vi "MQTT Publisher.vi"() -> ()   [LabVIEW 2021]
uses:
  <vilib>/LabVIEW Open Source Project/MQTT Control Packets/Control Packets/CONNECT/ConnectFlags -- cluster.ctl
  <vilib>/LabVIEW Open Source Project/MQTT Connection/MQTT_Base/Base Class/MQTT_Base.lvclass/MQTT_Base.ctl
  <vilib>/LabVIEW Open Source Project/Connection/Connection.TCP/Connection.TCP.lvclass
  C:/Program Files (x86)/National Instruments/LabVIEW 2021/vi.lib/LabVIEW Open Source Project/Connection/Connection/Connection.lvclass
  <vilib>/LabVIEW Open Source Project/MQTT Client/Client class/Client.lvclass
  C:/Program Files (x86)/National Instruments/LabVIEW 2021/vi.lib/LabVIEW Open Source Project/MQTT Connection/MQTT_Base/Base Class/MQTT_Base.lvclass
  <vilib>/LabVIEW Open Source Project/MQTT Control Packets/Control Packets/PUBLISH/PUBLISH.lvclass
  <vilib>/LabVIEW Open Source Project/MQTT Connection/MQTT_Base/Base Class/MQTT_Base.lvclass
  <vilib>/LabVIEW Open Source Project/MQTT Control Packets/Control Packets/CONNECT/CONNECT.lvclass
panel:
  out "Connected?":bool
  out "Published":bool
  in  "Topic":string
  out "Data Chart":dbl(graph)
  out "Data":dbl format="%#_4g"
  in  "Time Target (s)":dbl=1.0 format="%#_6ps"
  in  "remote port (1883)":u16=1883
  in  "address (localhost)":string="localhost"
  in  "STOP":bool
  # "MQTT Publisher"
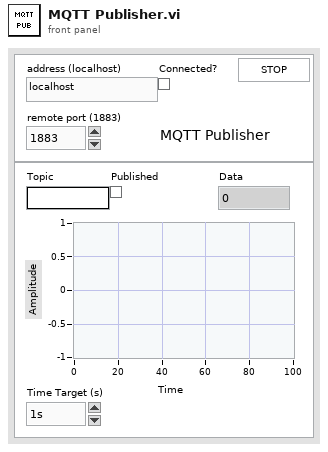
[diagram p1: front panel]
types:
  T1 = enum32{"Invalid", "Standard", "Closed", "Hidden", "Minimized", "Maximized"}
  T2 = enum32{"invalid app kind", "Development System", "Run Time System", "Student Edition", "Embedded LabVIEW", "Evaluation", "Custom"}
  T3 = typedef "MQTT_Control_Packets.lvlib/CONNECT.lvclass/ConnectFlags -- cluster.ctl" = cluster{"Reserved":bool, "Clean Session":bool, "Will Flag":bool, "Will QoS 1":bool, "Will QoS 2":bool, "Will Retain":bool, "Password Flag":bool, "User Name Flag":bool}
  T4 = cluster{"Will Topic":string, "Will Message":string, "Username":string, "Password":string}
  T5 = cluster{"Core":cluster{"Current VI Reference":refnum<vi>, "Close Panel on Exit?":bool}, "Connected?":bool, "Published?":bool, "Dummy Data":dbl}
  T6 = cluster{"Current VI Reference":refnum<vi>, "Close Panel on Exit?":bool}
  T7 = typedef "MQTT Base.lvlib/MQTT_Base.lvclass/Public Events -- cluster.ctl" = cluster{"Stop Event":refnum<user-event>, "Error Event":refnum<user-event>, "Inbound Message":refnum<user-event>}
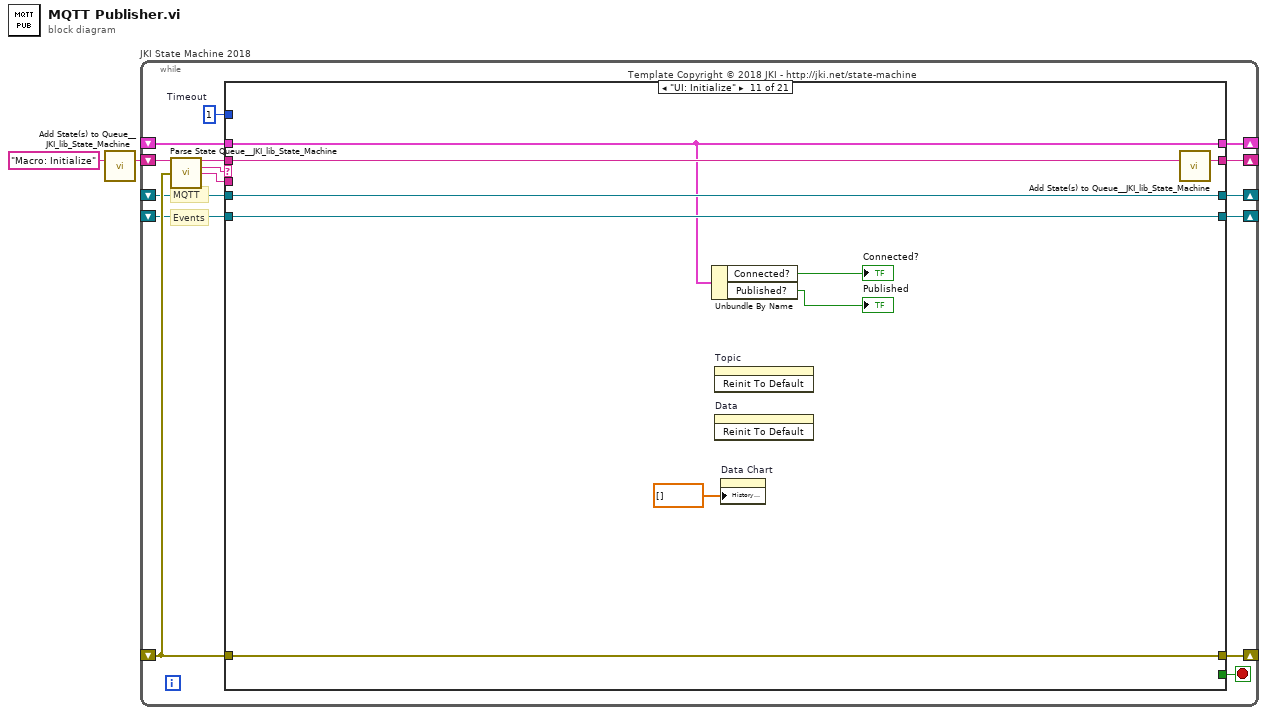
[diagram p0: block diagram]
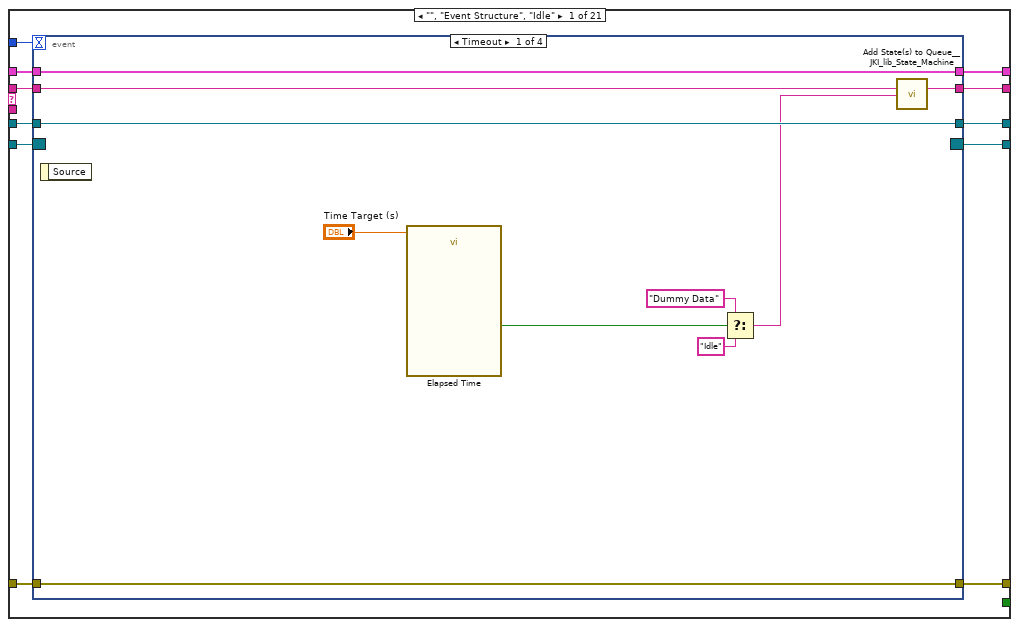
[diagram p2: hidden frame]
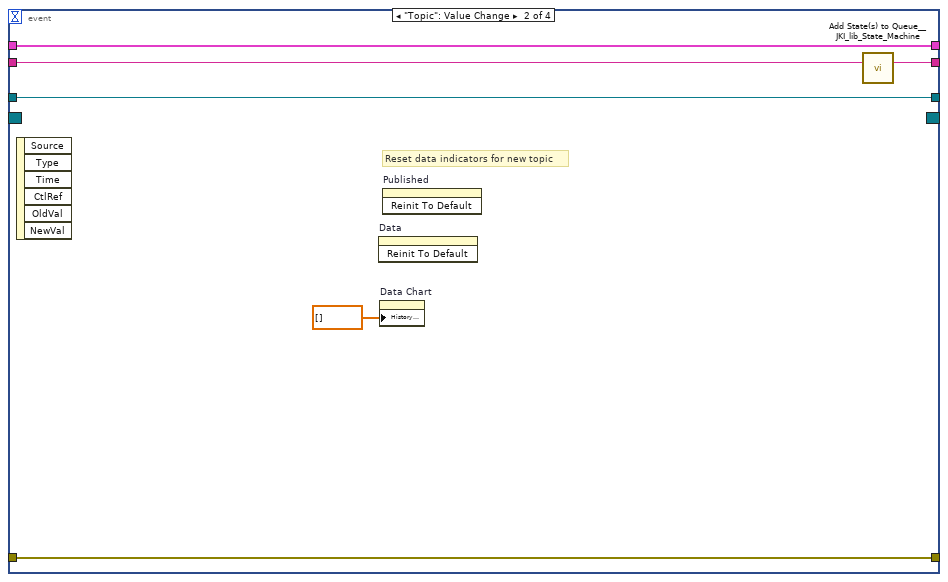
[diagram p3: hidden frame]
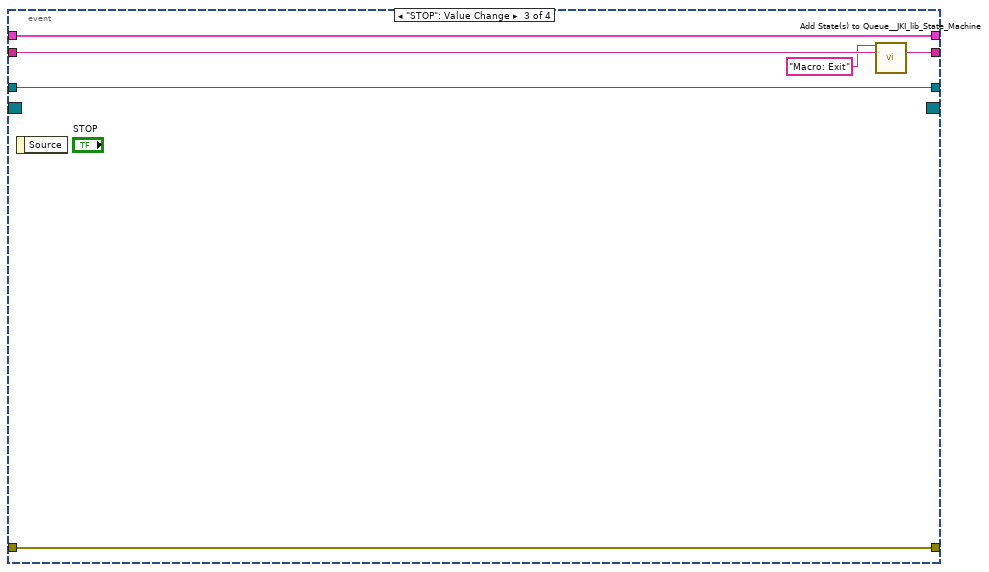
[diagram p4: hidden frame]
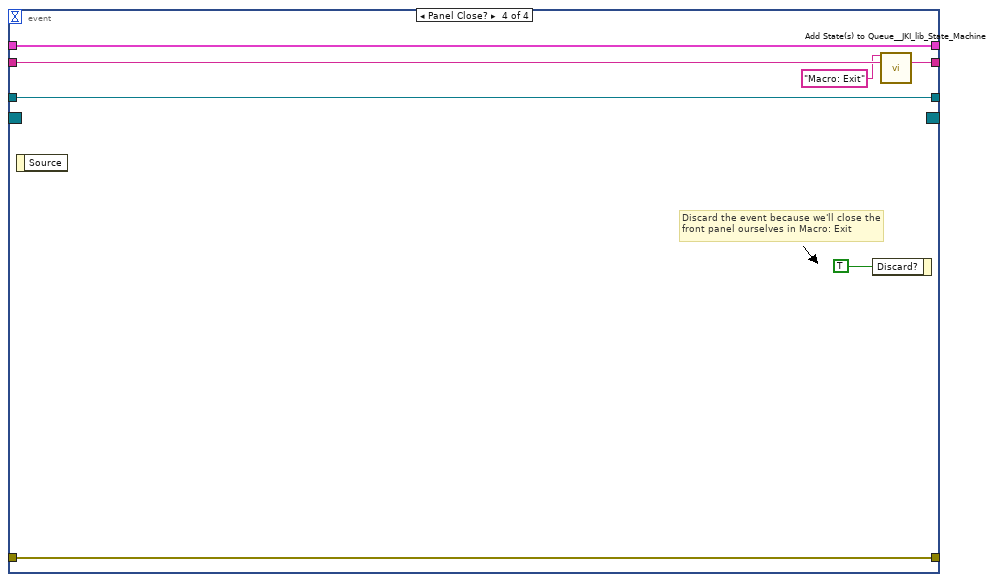
[diagram p5: hidden frame]
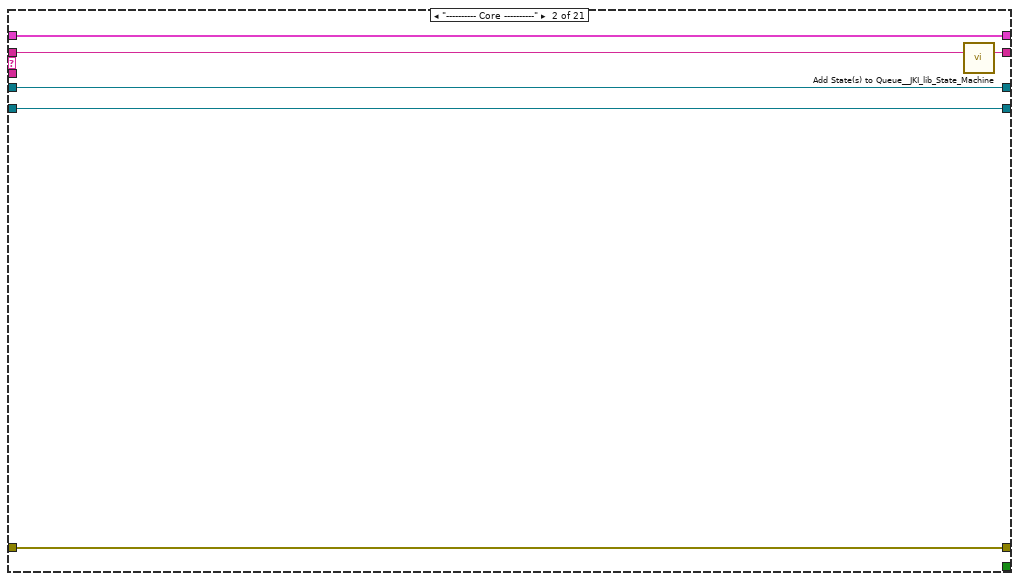
[diagram p6: hidden frame]
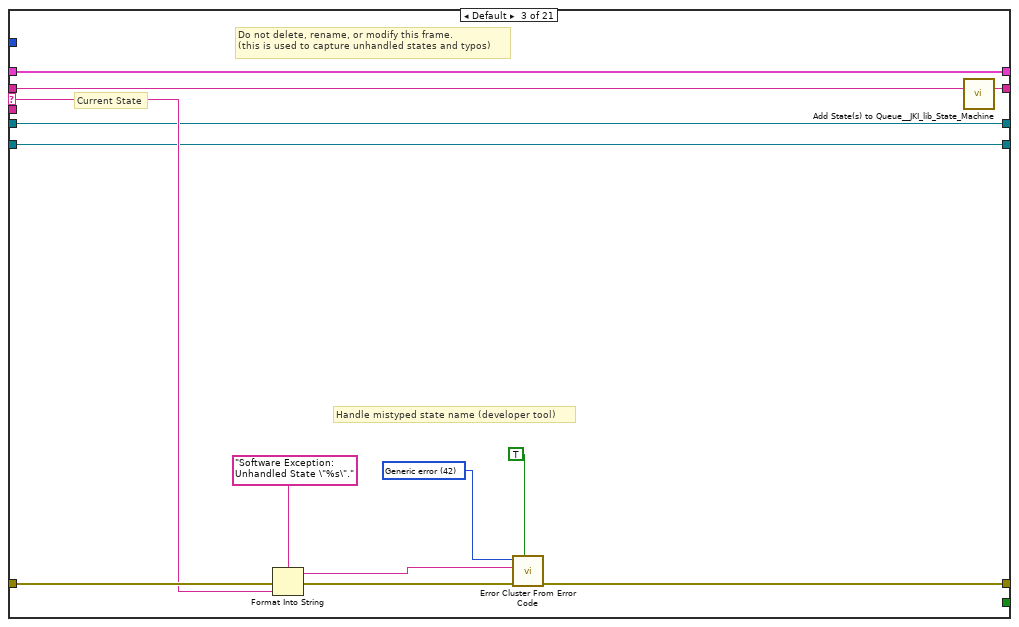
[diagram p7: hidden frame]
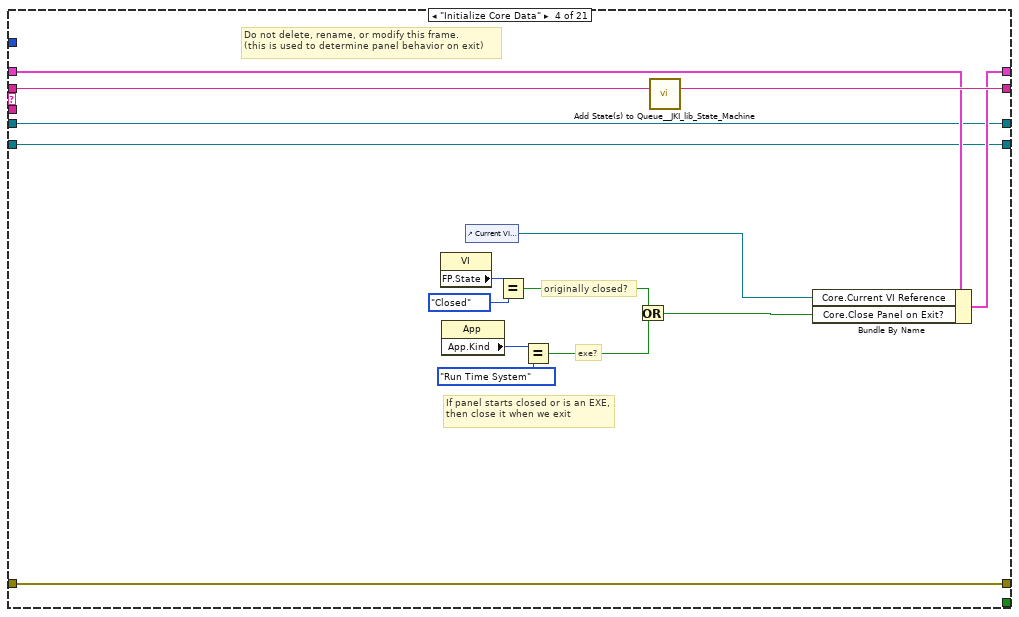
[diagram p8: hidden frame]
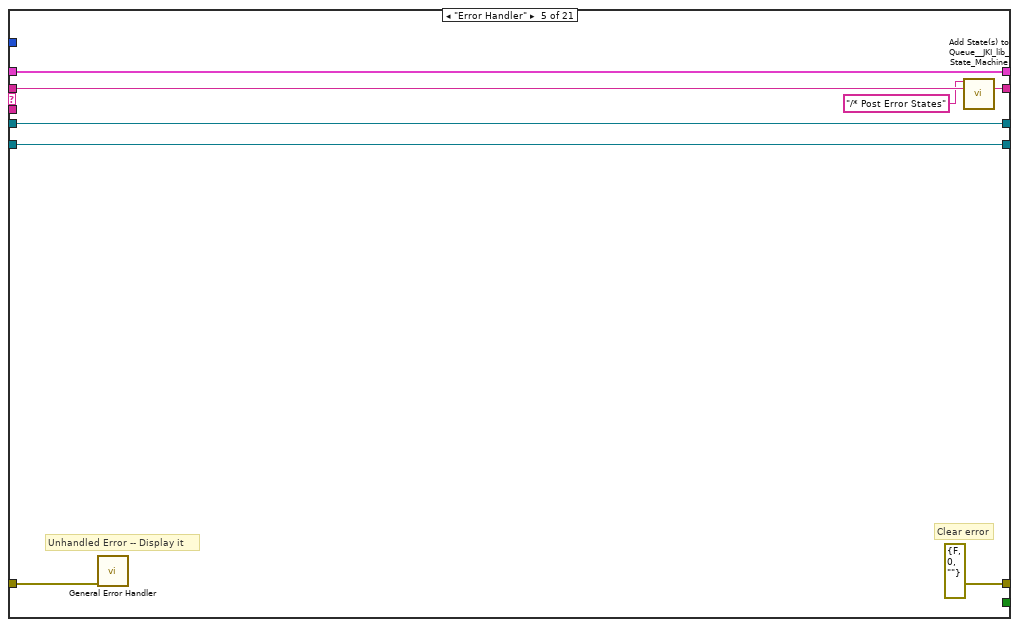
[diagram p9: hidden frame]
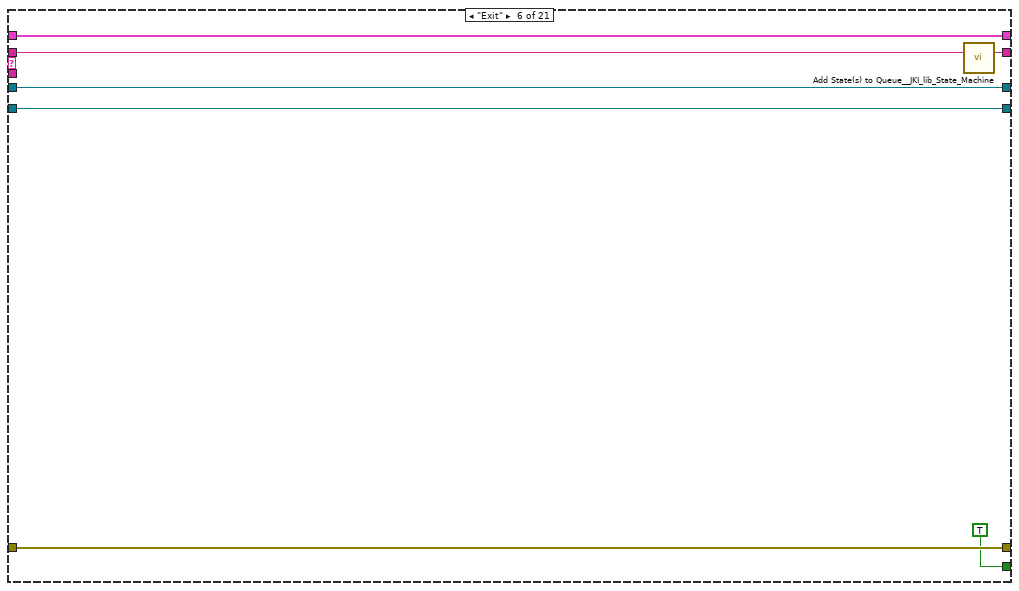
[diagram p10: hidden frame]
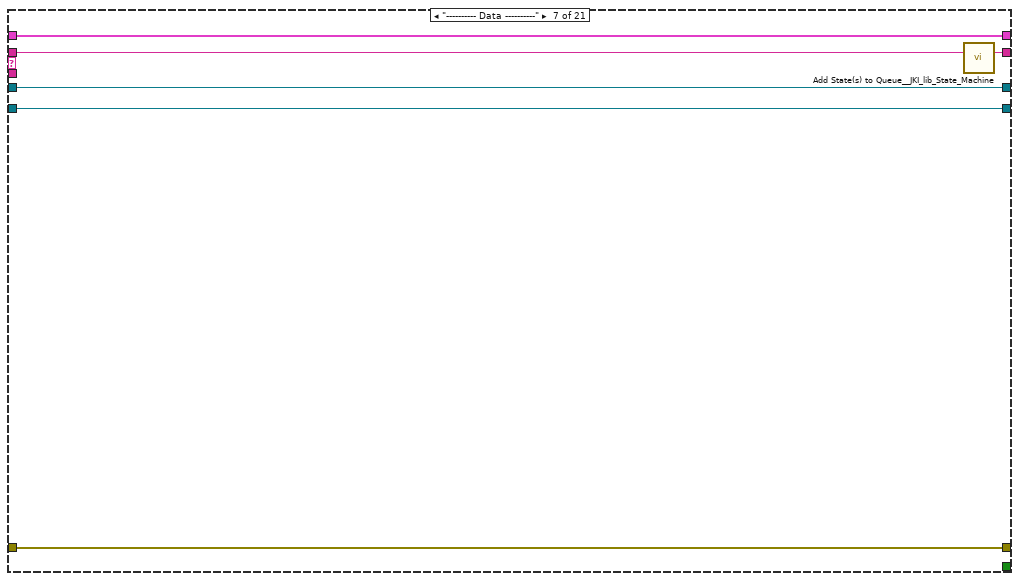
[diagram p11: hidden frame]
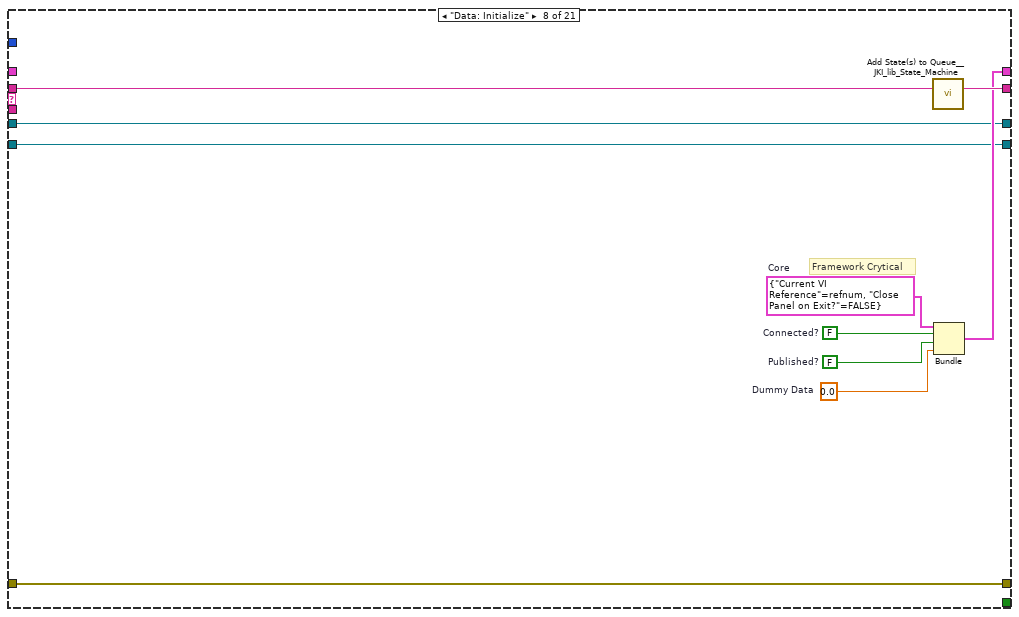
[diagram p12: hidden frame]
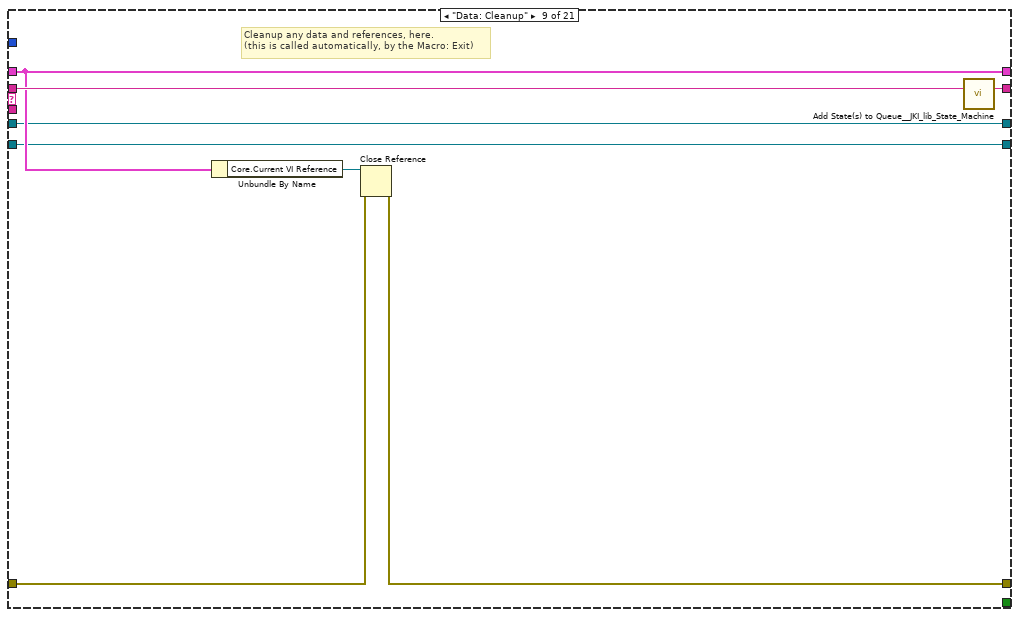
[diagram p13: hidden frame]
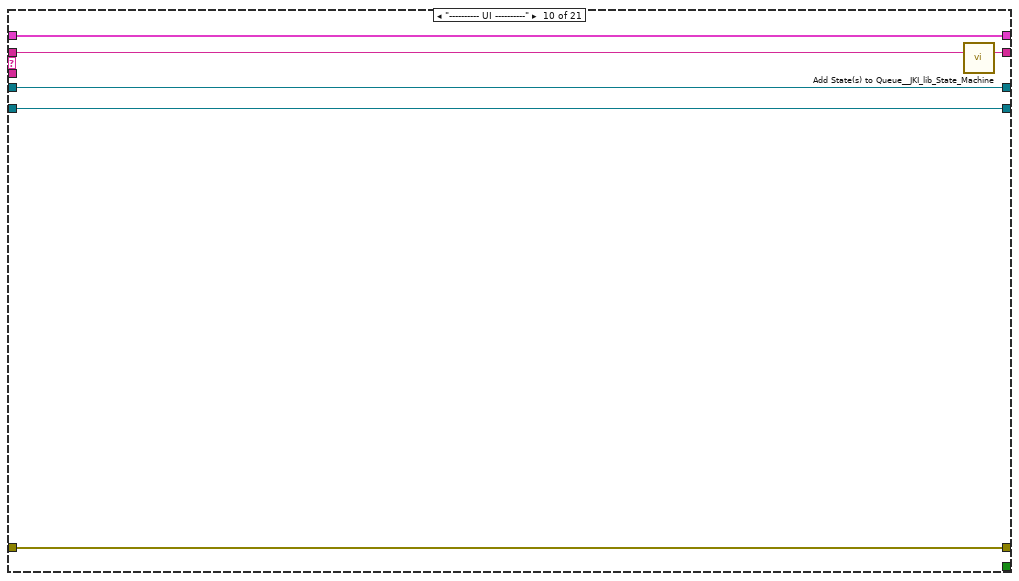
[diagram p14: hidden frame]
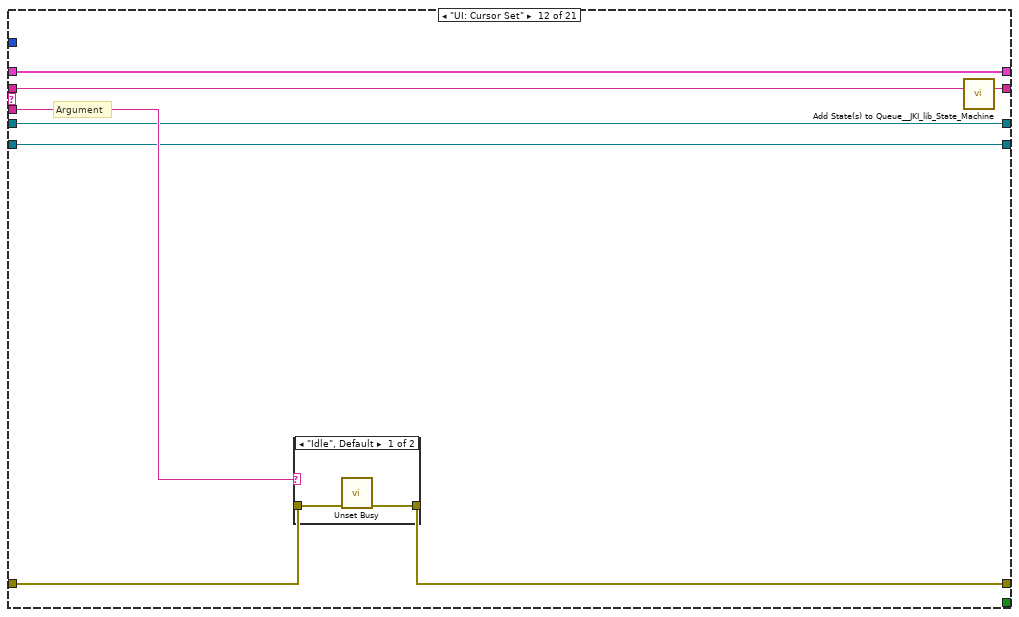
[diagram p15: hidden frame]
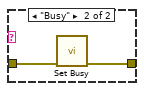
[diagram p16: hidden frame]
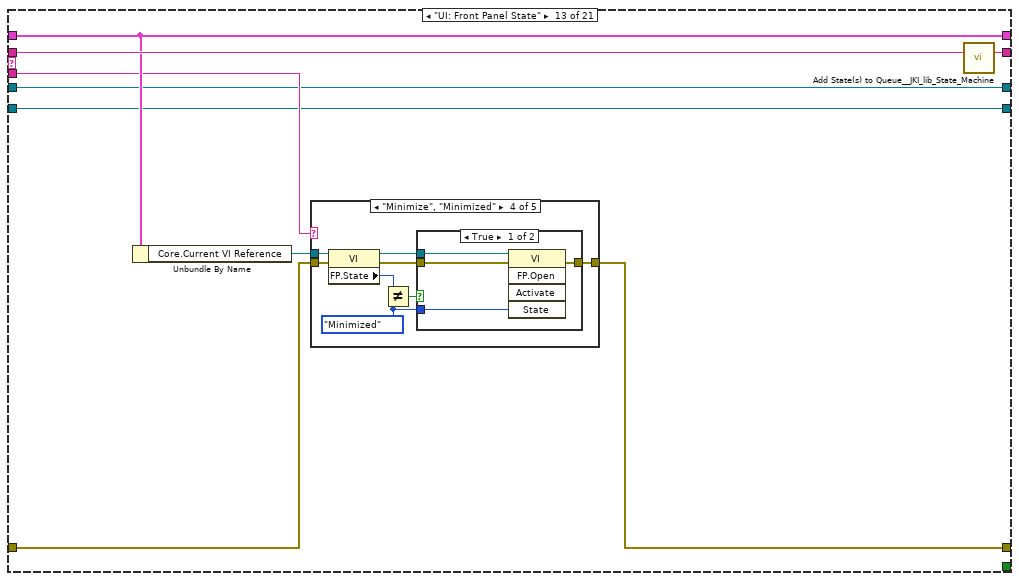
[diagram p17: hidden frame]
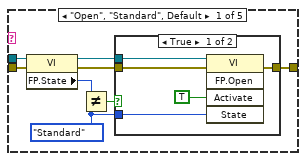
[diagram p18: hidden frame]
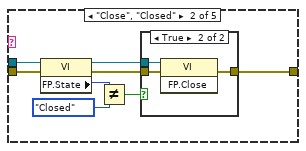
[diagram p20: hidden frame]
diagram:
  n1 = call <vilib>:"Add State(s) to Queue__JKI_lib_State_Machine.vi"("State(s) in (\"\")"="Macro: Initialize") -> ("States Out"=w2:string)  [unwired: 14 in]
  n2 = while "JKI State Machine 2018" {
    shift-right: [w10] -> _
    shift-left: _ -> [w9]
    shift-right: [w13] -> _
    shift-left: _ -> [w7]
    shift-right: [w12] -> _
    shift-left: w2 -> [w14]
    shift-right: [w6] -> _
    shift-left: _ -> [w5]
    shift-right: [w4] -> _
    shift-left: _ -> [w3]
    stop <- w11 stop-if-true
    w8 = 1  # Timeout
    # "Events"
    # "MQTT"
    # "Template Copyright © 2018 JKI - http://jki.net/state-machine"
    n3 = call <vilib>:"Parse State Queue__JKI_lib_State_Machine.vi"("State Queue"=w14, "Error In (no error)"=w7) -> ("Remaining States"=w16:string, "Current State"=w17:string, "Arguments"=w15:string)  [unwired: 11 in]
    n4 = case shown="\"UI: Initialize\"" w17 {
      selector: w17 -> [_ _ w66 _ _ _ _ _ _ _ _ _ _ _ _ _ _ _ _ _ _]
      tunnel: w16 -> [w28 w63 w70 w91 w99 w106 w112 w122 w130 w136 w145 w153 w166 w237 w244 w256 w262 w291 w304 w316 w327]
      tunnel: w15 -> [_ _ _ _ _ _ _ _ _ _ _ w148 w160 _ _ _ _ _ _ _ _]
      tunnel: w9 -> [w26 w60 w68 w84 w96 w104 w109 _ w125 w133 w140 w151 w162 w234 w241 w253 w259 w271 w295 w318 w324]
      tunnel: [w25 w61 w72 w88 errorcluster {"status"=FALSE, "code"=0, "source"=""} ("error out") w103 w110 w119 w126 w134 w143 w149 w163 w235 w242 w254 w260 w273 w297 w317 w328] -> w13
      tunnel: w7 -> [w24 w61 w71 w88 w95 w103 w110 w119 w127 w134 w143 w150 w164 w235 w242 w254 w260 w289 w300 w317 w328]
      tunnel: [w27 w62 w69 w90 w98 w105 w111 w121 w129 w135 w144 w152 w165 w236 w243 w255 w261 w290 w303 w315 w326] -> w12
      tunnel: [_ _ _ _ _ TRUE _ _ _ _ _ _ _ _ _ _ _ _ _ _ _] -> w11
      tunnel: [w23 w60 w68 w89 w96 w104 w109 w120 w125 w133 w140 w151 w162 w234 w241 w253 w259 w270 w294 w318 w323] -> w10
      tunnel: w8 -> [w22 _ _ _ _ _ _ _ _ _ _ _ _ _ _ _ _ _ _ _ _]
      tunnel: [w18 w58 w64 w77 w92 w100 w107 w116 w123 w131 w141 w146 w158 w232 w238 w245 w257 w288 w302 w320 w330] -> w6
      tunnel: w5 -> [w19 w58 w64 w77 w92 w100 w107 w116 w123 w131 w141 w146 w158 w232 w238 w245 w257 _ w302 w320 w330]
      tunnel: [w20 w59 w65 w78 w93 w101 w108 w117 w124 w132 w142 w147 w159 w233 w239 w246 w258 w272 w296 w319 w329] -> w4
      tunnel: w3 -> [w21 w59 w65 w78 w93 w101 w108 w117 w124 w132 w142 w147 w159 w233 w239 w246 w258 _ w301 w319 w329]
      frame "", "Event Structure", "Idle" {
        n5 = event shown="[0] Timeout" {
          selector: w19 -> [_ _ _ _]
          dyn-events: [_ _ _ _] -> w18
          timeout: w22 -> [_ _ _ _]
          tunnel: w28 -> [w38 w41 w50 w57]
          tunnel: [w37 w40 w49 w56] -> w27
          tunnel: w26 -> [w35 w43 w47 w54]
          tunnel: [w36 w44 w48 w55] -> w25
          tunnel: w24 -> [w36 w44 w48 w55]
          tunnel: [w35 w43 w47 w54] -> w23
          tunnel: w21 -> [w34 w42 w45 w51]
          tunnel: [w34 w42 w45 w51] -> w20
          event Timeout {
            n6 = event-data() -> ()  [unwired: 1 in, 1 out]
            n7 = call "Elapsed Time"("Time Target (s)"="Time Target (s)") -> ("Time has Elapsed"=w32:bool)  [unwired: 11 in, 7 out]
            n8 = Select(t="Dummy Data" ("State(s) at Back (\"\")"), s=w32, f="Idle" ("State(s) at Back (\"\")")) -> (s? t:f=w29:string)
            n9 = call <vilib>:"Add State(s) to Queue__JKI_lib_State_Machine.vi"("State(s) in (\"\")"=w38, "State(s) at Back (\"\")"=w29) -> ("States Out"=w37:string)  [unwired: 13 in]
          }
          event "Topic": Value Change {
            # "Reset data indicators for new topic"
            n10 = event-data() -> ()  [unwired: 1 in, 6 out]
            n11 = invoke on="Data" class="DigNum (strict)" method="Reinit To Default"() -> ()  [unwired: 3 in, 3 out]
            n12 = property on="Data Chart" class="WFChart (strict)"("History Data"=dbl[] []) -> ()  [unwired: 2 in, 2 out]
            n13 = invoke on="Published" class="Bool (strict)" method="Reinit To Default"() -> ()  [unwired: 3 in, 3 out]
            n14 = call <vilib>:"Add State(s) to Queue__JKI_lib_State_Machine.vi"("State(s) in (\"\")"=w41) -> ("States Out"=w40:string)  [unwired: 14 in]
          }
          event "STOP": Value Change {
            n15 = event-data() -> ()  [unwired: 1 in, 1 out]
            n16 = call <vilib>:"Add State(s) to Queue__JKI_lib_State_Machine.vi"("State(s) in Front (\"\")"="Macro: Exit", "State(s) in (\"\")"=w50) -> ("States Out"=w49:string)  [unwired: 13 in]
          }
          event Panel Close? {
            # "Discard the event because we'll close the front panel ourselves in Macro: Exit"
            n17 = event-data() -> ()  [unwired: 1 in, 1 out]
            n18 = event-data("Discard?"=TRUE) -> ()  [unwired: 1 in, 1 out]
            n19 = call <vilib>:"Add State(s) to Queue__JKI_lib_State_Machine.vi"("State(s) in Front (\"\")"="Macro: Exit", "State(s) in (\"\")"=w57) -> ("States Out"=w56:string)  [unwired: 13 in]
          }
        }
      }
      frame "---------- Core ----------" {
        n20 = call <vilib>:"Add State(s) to Queue__JKI_lib_State_Machine.vi"("State(s) in (\"\")"=w63) -> ("States Out"=w62:string)  [unwired: 14 in]
      }
      frame Default {
        w75 = 42 items=["No error", "Argument error", "Memory is full", "Out of zone", "End of file", "File already open", "Generic file I/O error", "File not found", "File permission error", "Disk is full", "Duplicate path", "Too many files open", "System feature not enabled", "Resource file not found", "Cannot add resource", "Resource not found", "Image not found", "Image memory error", "Pen does not exist", "Config type invalid", "Config token not found", "Config parse error", "Config memory error", "Bad external code format", "Bad external code offset", "External code not present", "Null window", "Destroy window error", "Null menu", "Print aborted", "Bad print record", "Print driver error", "Windows error during printing", "Memory error during printing", "Print dialog error", "Generic print error", "Invalid device refnum", "Device not found", "Device parameter error", "Device unit error", "Cannot open device", "Device call aborted", "Generic error", "Cancelled by user", "Object ID too low", "Object ID too high", "Object not in heap", "Unknown heap", "Unknown object (invalid DefProc)", "Unknown object (DefProc not in table)", "Message out of range", "Invalid (null) method", "Unknown message", "Manager call not supported", "Bad address", "Network operation in progress", "Network operation timed out", "Connection is busy", "Network attribute not supported", "Network error", "Address in use", "System out of memory", "Connection aborted", "Connection refused", "Not connected", "Already connected", "Connection closed", "Initialization error (interapplication manager)", "Bad occurrence", "Wait on unbound occurrence handler", "Occurrence queue overflow", "Datalog type conflict", "Unused", "Unrecognized type (interapplication manager)", "Memory corrupt", "Failed to make temporary DLL", "Old CIN version", "Drag socket not found", "Failed to load drop-object", "Failed to register OLE object", "Failed to release OLE object", "Format specifier type mismatch", "Unknown format specifier", "Too few format specifiers", "Too many format specifiers", "Scan failed", "Newer CIN version", "Error converting to variant", "Runtime menu error", "Password tampered", "Variant attribute not found", "Incompatible variant data type", "Event data is not available", "Event Store is not present", "Occurrence is not found", "Event Queue is not created", "Event info is not available", "Refnum passed is NULL", "Error retrieving Class GUID", "Error retrieving CoClass GUID", "Error retrieving TypeLib GUID.", "Bad built application magic bytes.", "Specific driver is different from the specific driver associated with the Logical Name.", "There is no session opened to the class driver.", "Max Error", "MAX - Error with config objects", "MAX - Error loading configuration", "MAX - Group not supported"]
        # "Current State"
        # "Do not delete, rename, or modify this frame.\n(this is used to capture unhandled states and typos)"
        # "Handle mistyped state name (developer tool)"
        n21 = Format Into String(format string="Software Exception: Unhandled State \"%s\"." ("message"), error in=w71, w66) -> (resulting string=w74:string, error out=w73:errorcluster)  [unwired: 1 in]
        n22 = call <vilib>:"Error Cluster From Error Code.vi"("show call chain? (False)"=TRUE, "error in (no error)"=w73, "error message (\"\")"=w74, "error code (0)"=w75) -> ("error out"=w72:errorcluster)  [unwired: 5 in]
        n23 = call <vilib>:"Add State(s) to Queue__JKI_lib_State_Machine.vi"("State(s) in (\"\")"=w70) -> ("States Out"=w69:string)  [unwired: 14 in]
      }
      frame "Initialize Core Data" {
        # "Do not delete, rename, or modify this frame.\n(this is used to determine panel behavior on exit)"
        # "originally closed?"
        # "exe?"
        # "If panel starts closed or is an EXE, then close it when we exit"
        n24 = property class="VI"() -> ("FP.State"=w81:T1)  [unwired: 2 in, 2 out]
        n25 = property class="App"() -> ("App.Kind"=w87:T2)  [unwired: 2 in, 2 out]
        n26 = control-ref of="Current VI Reference"() -> (w82:refnum<vi>)
        n27 = Equal?(x=w81, y=T1."Closed" ("Front Panel Window:State")) -> (x = y?=w79:bool)
        n28 = Equal?(x=w87, y=T2."Run Time System" ("Application:Kind")) -> (x = y?=w85:bool)
        n29 = Or(x=w79, y=w85) -> (x .or. y?=w83:bool)
        n30 = call <vilib>:"Add State(s) to Queue__JKI_lib_State_Machine.vi"("State(s) in (\"\")"=w91) -> ("States Out"=w90:string)  [unwired: 14 in]
        n31 = Bundle By Name(cluster=w84, "Core.Current VI Reference"=w82, "Core.Close Panel on Exit?"=w83) -> (w89:T5)
      }
      frame "Error Handler" {
        # "Unhandled Error -- Display it"
        # "Clear error"
        n32 = call <vilib>:"General Error Handler.vi"("error in (no error)"=w95) -> ()  [unwired: 10 in, 5 out]
        n33 = call <vilib>:"Add State(s) to Queue__JKI_lib_State_Machine.vi"("State(s) in Front (\"\")"="/* Post Error States", "State(s) in (\"\")"=w99) -> ("States Out"=w98:string)  [unwired: 13 in]
      }
      frame "Exit" {
        n34 = call <vilib>:"Add State(s) to Queue__JKI_lib_State_Machine.vi"("State(s) in (\"\")"=w106) -> ("States Out"=w105:string)  [unwired: 14 in]
      }
      frame "---------- Data ----------" {
        n35 = call <vilib>:"Add State(s) to Queue__JKI_lib_State_Machine.vi"("State(s) in (\"\")"=w112) -> ("States Out"=w111:string)  [unwired: 14 in]
      }
      frame "Data: Initialize" {
        w113 = FALSE  # Published?
        w115 = FALSE  # Connected?
        w114 = 0.0  # Dummy Data
        w118 = T6 {"Current VI Reference"=refnum, "Close Panel on Exit?"=FALSE}  # Core
        # "Framework Crytical"
        n36 = call <vilib>:"Add State(s) to Queue__JKI_lib_State_Machine.vi"("State(s) in (\"\")"=w122) -> ("States Out"=w121:string)  [unwired: 14 in]
        n37 = Bundle("Core"=w118, "Connected?"=w115, "Published?"=w113, "Dummy Data"=w114) -> (w120:T5)  [unwired: 1 in]
      }
      frame "Data: Cleanup" {
        # "Cleanup any data and references, here.\n(this is called automatically, by the Macro: Exit)"
        n38 = Unbundle By Name(w125) -> ("Core.Current VI Reference"=w128:refnum<vi>)
        n39 = Close Reference(reference=w128, error in (no error)=w127) -> (error out=w126:errorcluster)
        n40 = call <vilib>:"Add State(s) to Queue__JKI_lib_State_Machine.vi"("State(s) in (\"\")"=w130) -> ("States Out"=w129:string)  [unwired: 14 in]
      }
      frame "---------- UI ----------" {
        n41 = call <vilib>:"Add State(s) to Queue__JKI_lib_State_Machine.vi"("State(s) in (\"\")"=w136) -> ("States Out"=w135:string)  [unwired: 14 in]
      }
      frame "UI: Initialize" {
        n42 = Unbundle By Name(w140) -> ("Connected?"=→"Connected?":bool, "Published?"=→"Published":bool)
        n43 = invoke on="Topic" class="Str" method="Reinit To Default"() -> ()  [unwired: 3 in, 3 out]
        n44 = invoke on="Data" class="DigNum (strict)" method="Reinit To Default"() -> ()  [unwired: 3 in, 3 out]
        n45 = property on="Data Chart" class="WFChart (strict)"("History Data"=dbl[] []) -> ()  [unwired: 2 in, 2 out]
        n46 = call <vilib>:"Add State(s) to Queue__JKI_lib_State_Machine.vi"("State(s) in (\"\")"=w145) -> ("States Out"=w144:string)  [unwired: 14 in]
      }
      frame "UI: Cursor Set" {
        # "Argument"
        n47 = case shown="\"Idle\", Default" w148 {
          tunnel: w150 -> [w155 w157]
          tunnel: [w154 w156] -> w149
          frame "Idle", Default {
            n48 = call <vilib>:"Unset Busy.vi"("error in (no error)"=w155) -> ("error out"=w154:errorcluster)  [unwired: 10 in]
          }
          frame "Busy" {
            n49 = call <vilib>:"Set Busy.vi"("error in (no error)"=w157) -> ("error out"=w156:errorcluster)  [unwired: 9 in, 1 out]
          }
        }
        n50 = call <vilib>:"Add State(s) to Queue__JKI_lib_State_Machine.vi"("State(s) in (\"\")"=w153) -> ("States Out"=w152:string)  [unwired: 14 in]
      }
      frame "UI: Front Panel State" {
        n51 = Unbundle By Name(w162) -> ("Core.Current VI Reference"=w161:refnum<vi>)
        n52 = case shown="\"Minimize\", \"Minimized\"" w160 {
          tunnel: w164 -> [w172 w187 w198 w211 w224]
          tunnel: [w174 w188 w200 w213 w226] -> w163
          tunnel: w161 -> [w173 w185 w199 w212 w225]
          frame "Open", "Standard", Default {
            w167 = T1."Standard" ("State")
            n53 = property class="VI"(reference=w173, error in=w172) -> (reference out=w170:refnum<vi>, error out=w171:errorcluster, "FP.State"=w169:T1)
            n54 = Not Equal?(x=w169, y=w167) -> (x != y?=w168:bool)
            n55 = case shown="True" w168 {
              tunnel: [w178 w180] -> w174
              tunnel: w171 -> [w177 w180]
              tunnel: w170 -> [w176 _]
              tunnel: w167 -> [w175 _]
              frame True {
                n56 = invoke class="VI" method="FP.Open"(reference=w176, error in=w177, "Activate"=TRUE, "State"=w175) -> (error out=w178:errorcluster)  [unwired: 1 in, 4 out]
              }
              frame False {
              }
            }
          }
          frame "Close", "Closed" {
            n57 = property class="VI"(reference=w185, error in=w187) -> (reference out=w184:refnum<vi>, error out=w186:errorcluster, "FP.State"=w182:T1)
            n58 = Not Equal?(x=w182, y=T1."Closed" ("Front Panel Window:State")) -> (x != y?=w181:bool)
            n59 = case shown="True" w181 {
              tunnel: [w189 w192] -> w188
              tunnel: w186 -> [w189 w191]
              tunnel: w184 -> [_ w190]
              frame False {
              }
              frame True {
                n60 = invoke class="VI" method="FP.Close"(reference=w190, error in=w191) -> (error out=w192:errorcluster)  [unwired: 1 in, 2 out]
              }
            }
          }
          frame "Hidden", "Hide" {
            w193 = T1."Hidden" ("State")
            n61 = property class="VI"(reference=w199, error in=w198) -> (reference out=w196:refnum<vi>, error out=w197:errorcluster, "FP.State"=w195:T1)
            n62 = Not Equal?(x=w195, y=w193) -> (x != y?=w194:bool)
            n63 = case shown="True" w194 {
              tunnel: [w204 w205] -> w200
              tunnel: w197 -> [w203 w205]
              tunnel: w196 -> [w202 _]
              tunnel: w193 -> [w201 _]
              frame True {
                n64 = invoke class="VI" method="FP.Open"(reference=w202, error in=w203, "State"=w201) -> (error out=w204:errorcluster)  [unwired: 2 in, 4 out]
              }
              frame False {
              }
            }
          }
          frame "Minimize", "Minimized" {
            w206 = T1."Minimized" ("State")
            n65 = property class="VI"(reference=w212, error in=w211) -> (reference out=w209:refnum<vi>, error out=w210:errorcluster, "FP.State"=w208:T1)
            n66 = Not Equal?(x=w208, y=w206) -> (x != y?=w207:bool)
            n67 = case shown="True" w207 {
              tunnel: [w217 w218] -> w213
              tunnel: w210 -> [w216 w218]
              tunnel: w209 -> [w215 _]
              tunnel: w206 -> [w214 _]
              frame True {
                n68 = invoke class="VI" method="FP.Open"(reference=w215, error in=w216, "State"=w214) -> (error out=w217:errorcluster)  [unwired: 2 in, 4 out]
              }
              frame False {
              }
            }
          }
          frame "Maximize", "Maximized" {
            w219 = T1."Maximized" ("State")
            n69 = property class="VI"(reference=w225, error in=w224) -> (reference out=w222:refnum<vi>, error out=w223:errorcluster, "FP.State"=w221:T1)
            n70 = Not Equal?(x=w221, y=w219) -> (x != y?=w220:bool)
            n71 = case shown="True" w220 {
              tunnel: [w230 w231] -> w226
              tunnel: w223 -> [w229 w231]
              tunnel: w222 -> [w228 _]
              tunnel: w219 -> [w227 _]
              frame True {
                n72 = invoke class="VI" method="FP.Open"(reference=w228, error in=w229, "State"=w227) -> (error out=w230:errorcluster)  [unwired: 2 in, 4 out]
              }
              frame False {
              }
            }
          }
        }
        n73 = call <vilib>:"Add State(s) to Queue__JKI_lib_State_Machine.vi"("State(s) in (\"\")"=w166) -> ("States Out"=w165:string)  [unwired: 14 in]
      }
      frame "---------- Macro ----------" {
        n74 = call <vilib>:"Add State(s) to Queue__JKI_lib_State_Machine.vi"("State(s) in (\"\")"=w237) -> ("States Out"=w236:string)  [unwired: 14 in]
      }
      frame "Macro: Initialize" {
        n75 = call <vilib>:"Add State(s) to Queue__JKI_lib_State_Machine.vi"("State(s) in Front (\"\")"="Data: Initialize\nInitialize Core Data\nMQTT: Initialize\nUI: Initialize\nUI: Front Panel State >> Open", "State(s) in (\"\")"=w244) -> ("States Out"=w243:string)  [unwired: 13 in]
      }
      frame "Macro: Exit" {
        n76 = Unbundle By Name(w253) -> ("Core.Close Panel on Exit?"=w252:bool)
        n77 = Select(t="UI: Front Panel State >> Close", s=w252, f="") -> (s? t:f=w249:string)
        n78 = call <vilib>:"Add State(s) to Queue__JKI_lib_State_Machine.vi"("State(s) in (\"\")"=w249, "State(s) at Back (\"\")"="Data: Cleanup\nExit") -> ("States Out"=w247:string)  [unwired: 13 in]
        n79 = call <vilib>:"Add State(s) to Queue__JKI_lib_State_Machine.vi"("State(s) in Front (\"\")"=w247, "State(s) in (\"\")"=w256) -> ("States Out"=w255:string)  [unwired: 13 in]
      }
      frame "---------- MQTT Broker ----------" {
        n80 = call <vilib>:"Add State(s) to Queue__JKI_lib_State_Machine.vi"("State(s) in (\"\")"=w262) -> ("States Out"=w261:string)  [unwired: 14 in]
      }
      frame "MQTT: Initialize" {
        # "Exit on fail"
        # "Connect"
        n81 = call <vilib>:"Configure TCP Connection.vi"("error in (no error)"=w289, "remote port (80)"="remote port (1883)", "address (localhost)"="address (localhost)") -> ("error out"=w284:errorcluster, "Connection.TCP"=w283:refnum<class "Connection.TCP.lvclass">)  [unwired: 7 in]
        n82 = call <vilib>:"Create MQTT Client.vi"("error in (no error)"=w284, "Connection Configuration"=w283) -> ("error out"=w281:errorcluster, "Client out"=w282:refnum<class "Client.lvclass">)  [unwired: 8 in]
        n83 = call <vilib>:"Read MQTT Public Events.vi"("error in (no error)"=w281, "MQTT_Base in"=w282) -> ("error out"=w279:errorcluster, "MQTT Public Events"=w280:T7, "MQTT_Base out"=w278:refnum<class "Client.lvclass">)  [unwired: 7 in]
        n84 = register-events(error in=w279, w280) -> (reference out=w288:refnum<event-registration>, error out=w287:errorcluster)  [unwired: 1 in]
        n85 = call <vilib>:"Start.vi"("error in (no error)"=w287, "MQTT_Base in"=w278) -> ("error out"=w276:errorcluster, "MQTT_Base out"=w277:refnum<class "Client.lvclass">)  [unwired: 7 in, 1 out]
        n86 = call <vilib>:"Connect to Server.vi"("Connect Flags"=T3 {"Reserved"=FALSE, "Clean Session"=TRUE, "Will Flag"=FALSE, "Will QoS 1"=FALSE, "Will QoS 2"=FALSE, "Will Retain"=FALSE, "Password Flag"=TRUE, "User Name Flag"=TRUE}, "Payload"=T4 {"Will Topic"="", "Will Message"="", "Username"="username", "Password"="password"}, "error in (no error)"=w276, "Client in"=w277) -> ("error out"=w274:errorcluster, "Client out"=w275:refnum<class "Client.lvclass">)  [unwired: 4 in, 2 out]
        n87 = call <vilib>:"isSessionConnected.vi"("error in (no error)"=w274, "MQTT_Base in"=w275) -> ("error out"=w273:errorcluster, "Connected?"=w268:bool, "MQTT_Base out"=w272:refnum<class "Client.lvclass">)  [unwired: 7 in]
        n88 = Bundle By Name(cluster=w271, "Connected?"=w268, "Published?"=FALSE) -> (w270:T5)
        n89 = Select(t="", s=w268, f="Macro: Exit" ("State(s) at Back (\"\")")) -> (s? t:f=w266:string)
        n90 = call <vilib>:"Add State(s) to Queue__JKI_lib_State_Machine.vi"("State(s) in (\"\")"=w291, "State(s) at Back (\"\")"=w266) -> ("States Out"=w290:string)  [unwired: 13 in]
      }
      frame "MQTT: Publish Data" {
        n91 = call <vilib>:"isSessionConnected.vi"("error in (no error)"=w300, "MQTT_Base in"=w301) -> ("error out"=w298:errorcluster, "Connected?"=w293:bool, "MQTT_Base out"=w299:refnum<class "Client.lvclass">)  [unwired: 7 in]
        n92 = case shown="True" w293 {
          tunnel: w299 -> [w305 w313]
          tunnel: w298 -> [w306 w312]
          tunnel: w295 -> [_ w314]
          tunnel: [_ w309] -> w292
          tunnel: [w306 w308] -> w297
          tunnel: [w305 w307] -> w296
          frame False {
          }
          frame True {
            n93 = Unbundle By Name(w314) -> ("Dummy Data"=w310:dbl)
            n94 = call <vilib>:"Publish.vi"("error in (no error)"=w312, "Payload"=w310, "Topic Name (empty: Payload name)"="Topic", "Client in"=w313) -> ("error out"=w308:errorcluster, "Published"=w309:bool, "Client out"=w307:refnum<class "Client.lvclass">)  [unwired: 5 in]
          }
        }
        n95 = property on="Connected?" class="Bool (strict)"("Value"=w293) -> ()  [unwired: 2 in, 2 out]
        n96 = property on="Published" class="Bool (strict)"("Value"=w292) -> ()  [unwired: 2 in, 2 out]
        n97 = Bundle By Name(cluster=w295, "Connected?"=w293, "Published?"=w292) -> (w294:T5)
        n98 = call <vilib>:"Add State(s) to Queue__JKI_lib_State_Machine.vi"("State(s) in (\"\")"=w304) -> ("States Out"=w303:string)  [unwired: 14 in]
      }
      frame "---------- Dummy Data ----------" {
        n99 = call <vilib>:"Add State(s) to Queue__JKI_lib_State_Machine.vi"("State(s) in (\"\")"=w316) -> ("States Out"=w315:string)  [unwired: 14 in]
      }
      frame "Dummy Data" {
        # "Generate a sine wave"
        n100 = for {
          N: 1 -> [_]
          shift-right: [w331] -> _
          shift-left: _ -> [w332]
          tunnel: [w334] -> w321
          n101 = Add(x=0.1, y=w332) -> (x+y=w331:dbl)
          n102 = Sine(x=w331) -> (sin(x)=w334:dbl)
        }
        "Data" <- w321
        "Data Chart" <- w321
        n103 = Bundle By Name(cluster=w324, "Dummy Data"=w321) -> (w323:T5)
        n104 = call <vilib>:"Add State(s) to Queue__JKI_lib_State_Machine.vi"("State(s) in (\"\")"=w327, "State(s) at Back (\"\")"="MQTT: Publish Data" ("State(s) at Back (\"\")")) -> ("States Out"=w326:string)  [unwired: 13 in]
      }
    }
  }
